vi "Save_Time_Traces.vi"() -> (5 "Plug in titles":string[](array[string]), 7 "Plug in values":string[](array[string]))   [LabVIEW 2022 SP3]
uses:
  Controls/File Header mode.ctl
  Controls/Average_Interpolate.ctl
  Globals/Meas_global.vi
panel:
  in  "Mode":T1
  in  "Headers":T2=enum."Headers in All files"
  in  "Each instrument in separate file":bool
  in  "Resampling Rate Hz in":dbl=100.0
  in  "Use Fixed Resampling Rate":bool
  in  "Channels to Save":T3(ring)=enum."All channels except Sync"
  in  "File Extension":string=".txt"
  in  "Put each block into separate file":bool
  in  "Leave space between blocks?":bool
  in  "Precision":i16=2
  in  "Data to save":i32[](array[ring]) items=["Gen (D)", "RV (Lift)", "RV (Pitch)", "RV (Drag)", "RV (Side-Force)", "RV (Yaw)", "RV (Roll)", "RZ (P1)", "RZ (P2)", "RZ (P3)", "RZ (P4)", "RZ (P5)", "RZ (P6)", "RZ (P7)", "RZ (P8)", "RZ (P9)", "RZ (P10)", "RZ (P11)", "RZ (P12)", "RZ (P13)", "RZ (P14)", "RZ (P15)", "RZ (P16)", "RZ (P21)", "RZ (P22)", "RZ (P23)", "RZ (P24)", "RZ (P25)", "RZ (P26)", "RZ (P27)", "RZ (P28)", "RZ (P29)", "RZ (P30)", "RZ (P31)", "RZ (P32)", "RV (Lift_Av)", "RV (Pitch_Av)", "RV (Drag_Av)", "RV (Side-Force_Av)", "RV (Yaw_Av)", "RV (Roll_Av)", "Save Nothing"]
  in  "Separation Character":enum16{"Tab", "Comma"}(ring)
  # "Run this VI to update the channel names"
  # "You Must have selected the \"Save Data\" option on the \nMeasurement Program for this vi to save time traces"
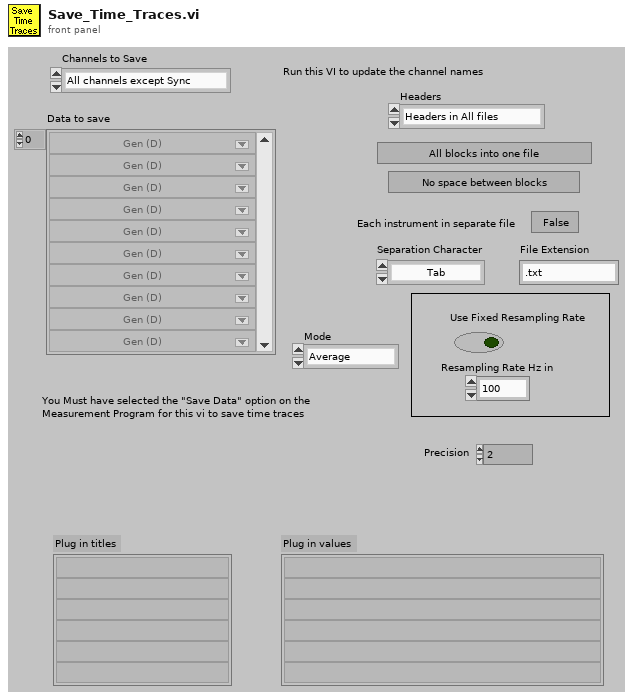
[diagram p1: front panel]
types:
  T1 = typedef "Average_Interpolate.ctl" = enum16{"Average", "Interpolate"}
  T2 = typedef "File Header mode.ctl" = enum16{"No Headers", "Headers in All files", "Separate Header File"}
  T3 = enum16{"Selected", "All channels except Sync", "All Channels"}
  T4 = typedef "Analysis_info_cluster.ctl" = cluster{"Colour":u32, "Inst type":T5, "Inst name":string, "Symbol":string, "Code name":string, "Extra Info":string, "Inst Array":T6, "Extra Titles":string[], "Extra Values":string[], "U":dbl, "u^2":dbl, "u^3":dbl, "u^4":dbl, "Skew_u":dbl, "Kurt_u":dbl, "Sd Error in Mean":dbl, "% u'/U":dbl, "X":dbl, "Y":dbl, "Z":dbl, "Timescale integral Estimate":dbl, "Sd Error in Variance":dbl, "Calib File":path, "Calib Constants":dbl[], "Output Position":bool, "Stats":enum16{"None", "Basic", "Full"}, "Av Sampling Rate":dbl, "Av No of Samples":dbl, "Total Meas Time (s)":dbl, "ADAM Ch Name":string, "Max value":dbl, "Min value":dbl, "Req Sample Rate Hz":dbl, "Sync Delay Time (s)":dbl, "Ch No":i16, "Device":string, "Use Latest Calib":bool, "Port":string, "Metadata Ch Names":string[], "Metadata Ch Values":string[], "Label":string}
  T5 = typedef "Inst_type.ctl" = enum16{"Raw voltage", "Raw with zero offsetting", "Propeller anemometer", "Pressure Transducer", "Pitot-static tube", "Hot wire", "Cross wire 1", "Cross wire 2", "Generic Linear", "Generic Polynomial", "Generic BackPoly", "Fast FID", "Thermocouple", "Cold wire", "Pulsed Wire", "LDA Vel", "LDA Tran time", "LDA Arr time", "Microphone"}
  T6 = typedef "Instrument_Array.ctl" = enum16{"PWA", "LDA", "Analogue"}
  T7 = enum16{"Save no data", "Save data in new files", "Save data in existing files"}
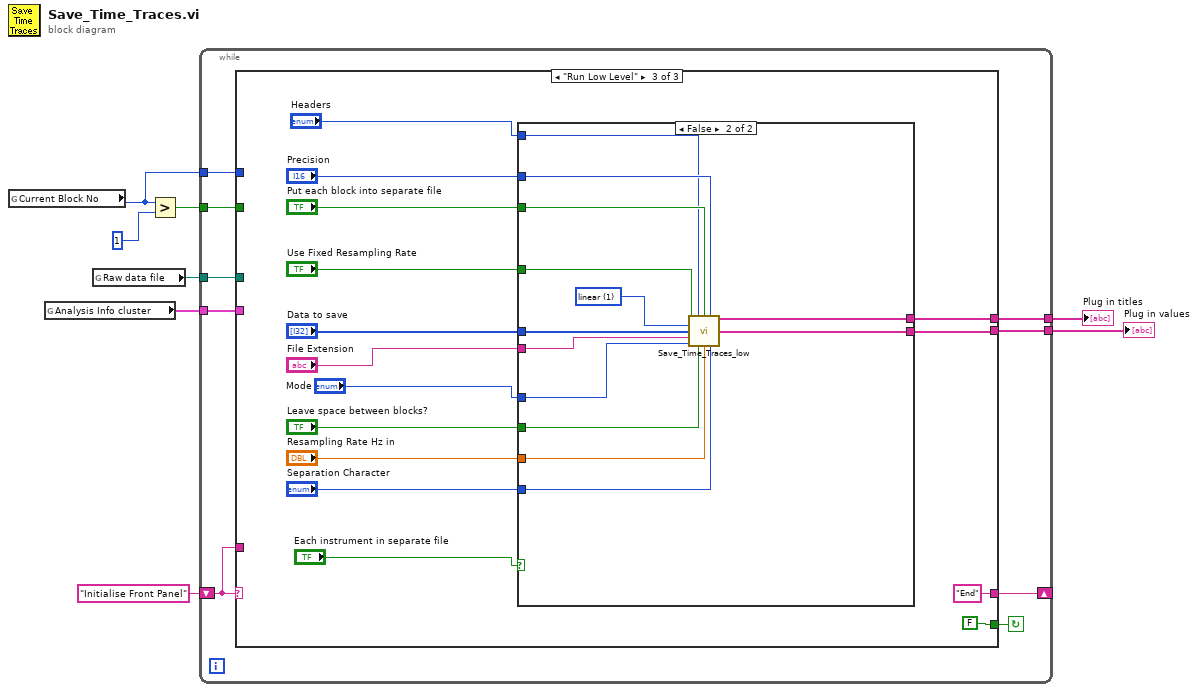
[diagram p0: block diagram]
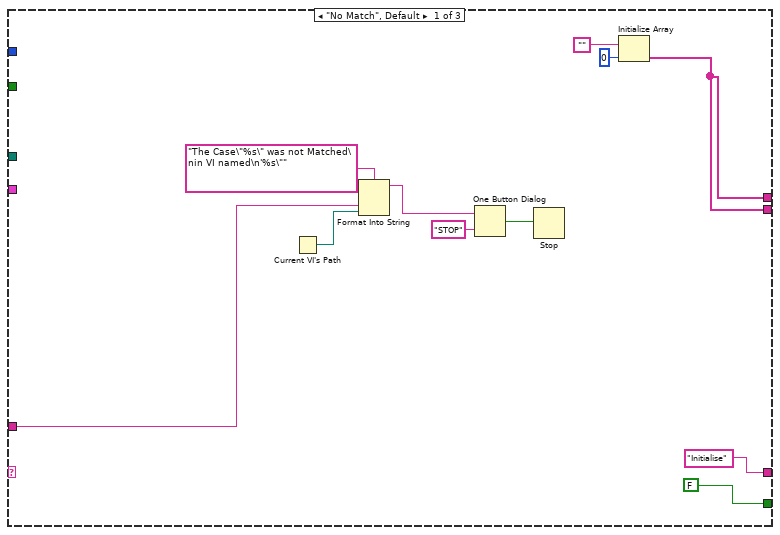
[diagram p2: hidden frame]
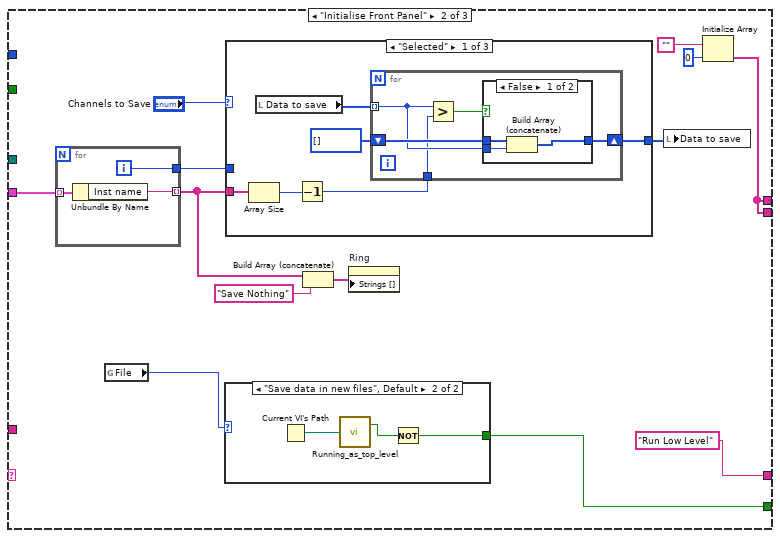
[diagram p3: hidden frame]
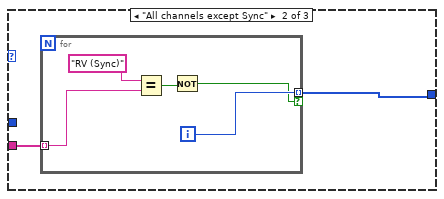
[diagram p5: hidden frame]
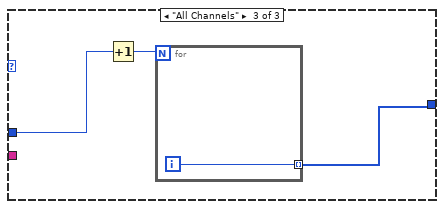
[diagram p6: hidden frame]
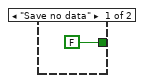
[diagram p7: hidden frame]
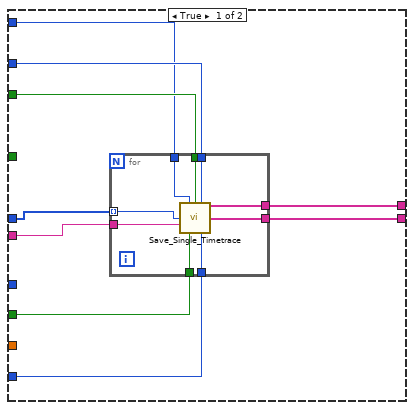
[diagram p8: hidden frame]
diagram:
  n1 = global read "Meas_global.vi" "Current Block No"() -> (w4:i32)
  n2 = global read "Meas_global.vi" "Analysis Info cluster"() -> (w3:T4[])
  n3 = global read "Meas_global.vi" "Raw data file"() -> (w7:path)
  n4 = Greater?(x=w4, y=1) -> (0:w5:bool)
  n5 = while {
    shift-left: "Initialise Front Panel" -> [w15]
    shift-right: [w16] -> _
    tunnel: w7 -> [w14]
    tunnel: w5 -> [w13]
    tunnel: w4 -> [w12]
    tunnel: w3 -> [w11]
    tunnel: [w10] -> w2
    tunnel: [w9] -> w1
    stop <- w17 continue-if-true
    n6 = case shown="\"Run Low Level\"" w15 {
      tunnel: [FALSE w34 FALSE] -> w17
      tunnel: ["Initialise" "Run Low Level" ("t") "End" ("t")] -> w16
      tunnel: w15 -> [w23 _ _]
      tunnel: w14 -> [_ _ _]
      tunnel: w13 -> [_ _ _]
      tunnel: w12 -> [_ _ _]
      tunnel: w11 -> [_ w41 _]
      tunnel: [w18 w29 w80] -> w10
      tunnel: [w18 w29 w81] -> w9
      frame "No Match", Default {
        n7 = Current VI's Path() -> (path=w22:path)
        n8 = Format Into String(format string="The Case\"%s\" was not Matched\nin VI named\n'%s\"" ("Format String"), w23, w22) -> (resulting string=w26:string)  [unwired: 2 in, 1 out]
        n9 = One Button Dialog(message=w26, button name ("OK")="STOP") -> (true=w24:bool)
        n10 = Stop(stop? (T)=w24) -> ()
        n11 = Initialize Array("", 0) -> (w18:string[])
      }
      frame "Initialise Front Panel" {
        n12 = for {
          tunnel: w41 -> [w74] mode=indexing
          tunnel: [w73] -> w37 mode=indexing
          tunnel: [w72] -> w32
          i -> [w72]
          n13 = Unbundle By Name(w74) -> ("Inst name"=w73:string)
        }
        n14 = global read "Meas_global.vi" "File"() -> (w35:T7)
        n15 = case shown="\"Save data in new files\", Default" w35 {
          tunnel: [FALSE w69] -> w34
          frame "Save no data" {
          }
          frame "Save data in new files", Default {
            n16 = Current VI's Path() -> (path=w70:path)
            n17 = call "Running_as_top_level.vi"("Vi path name"=w70) -> ("Top Level"=w71:bool)  [unwired: 1 out]
            n18 = Not(x=w71) -> (.not. x?=w69:bool)
          }
        }
        n19 = case shown="\"Selected\"" "Channels to Save" {
          tunnel: [w45 w58 w65] -> w40
          tunnel: w37 -> [w42 w57 _]
          tunnel: w32 -> [_ _ w66]
          frame "Selected" {
            n20 = Array Size(array=w42) -> (size(s)=w44:i32)
            n21 = local read "Data to save"() -> (w47:i32[])
            n22 = Decrement(x=w44) -> (x-1=w43:i32)
            n23 = for {
              tunnel: w47 -> [w49] mode=indexing
              shift-right: [w50] -> w45
              shift-left: i32[] [] -> [w51]
              tunnel: w43 -> [w48]
              n24 = Greater?(x=w49, y=w48) -> (0:w52:bool)
              n25 = case shown="False" w52 {
                tunnel: w51 -> [w55 w56]
                tunnel: [w54 w56] -> w50
                tunnel: w49 -> [w53 _]
                frame False {
                  n26 = Build Array (concatenate)(w55, w53) -> (w54:i32[])
                }
                frame True {
                }
              }
            }
          }
          frame "All channels except Sync" {
            n27 = for {
              tunnel: [w63] -> w58 mode=indexing if=w59
              tunnel: w57 -> [w62] mode=indexing
              i -> [w63]
              n28 = Equal?(x="RV (Sync)", y=w62) -> (x = y?=w60:bool)
              n29 = Not(x=w60) -> (.not. x?=w59:bool)
            }
          }
          frame "All Channels" {
            n30 = Increment(x=w66) -> (x+1=w64:i32)
            n31 = for {
              N: w64 -> [_]
              tunnel: [w67] -> w65 mode=indexing
              i -> [w67]
            }
          }
        }
        n32 = Build Array (concatenate)(w37, "Save Nothing") -> (w38:string[])
        n33 = property on="Ring" class="Ring (strict)"("Strings []"=w38) -> ()  [unwired: 2 in, 2 out]
        n34 = local write "Data to save"(w40) -> ()
        n35 = Initialize Array("", 0) -> (w29:string[])
      }
      frame "Run Low Level" {
        n36 = case shown="False" "Each instrument in separate file" {
          tunnel: "Put each block into separate file" -> [w98 w120]
          tunnel: "Precision" -> [w97 w119]
          tunnel: "Leave space between blocks?" -> [w96 w118]
          tunnel: "Data to save" -> [w91 w117]
          tunnel: "File Extension" -> [w95 w116]
          tunnel: "Mode" -> [_ w115]
          tunnel: "Separation Character" -> [w94 w114]
          tunnel: [w93 w113] -> w81
          tunnel: [w92 w112] -> w80
          tunnel: "Resampling Rate Hz in" -> [_ w111]
          tunnel: "Use Fixed Resampling Rate" -> [_ w110]
          tunnel: "Headers" -> [w90 w109]
          frame True {
            n37 = for {
              tunnel: w98 -> [w107]
              tunnel: w97 -> [w106]
              tunnel: w96 -> [w105]
              tunnel: w95 -> [w104]
              tunnel: w94 -> [w103]
              tunnel: [w102] -> w93
              tunnel: [w101] -> w92
              tunnel: w91 -> [w100] mode=indexing
              tunnel: w90 -> [w99]
              n38 = call "Save_Single_Timetrace.vi"("Headers"=w99, "Put each block into separate file"=w107, "Precision"=w106, "Index"=w100, "File Extension"=w104, "Leave space between blocks?"=w105, "Separation Character"=w103) -> ("Plug in titles"=w102:string[], "Plug in values"=w101:string[])  [unwired: 7 in]
            }
          }
          frame False {
            w108 = 1 items=["nearest", "linear", "spline", "cubic Hermite", "Lagrange"] ("method")
            n39 = call "Save_Time_Traces_low.vi"("Use Fixed Resampling Rate"=w110, "Headers"=w109, "Put each block into separate file"=w120, "Precision"=w119, "method"=w108, "Data to save"=w117, "File Extension"=w116, "Mode"=w115, "Leave space between blocks?"=w118, "Resampling Rate Hz in"=w111, "Separation Character"=w114) -> ("Plug in titles"=w113:string[], "Plug in values"=w112:string[])  [unwired: 3 out]
          }
        }
      }
    }
  }
  "Plug in values" <- w2
  "Plug in titles" <- w1
